vi "SRV_Motors Config GUI.vi"(11 "Motors Config File Path in":path) -> (0 "error out":errorcluster, 1 "Cancelled?":bool, 3 "Motor Config Filepath":path)   [LabVIEW 2014]
doc: "A Producer-Consumer two-loop state machine template. This template uses the LPD Command Queues to drive its execution.\n\nThere are several advantages such as:\n- convenient error state control\n- the ability to pass data between states/loops/VIs via a variant\n- command history which is extremely valuable in troubleshooting when an error occurs\n\n\nAuthor: Mike Schultz\n\nLogicPD, Inc\nwww.logicpd.com"
uses:
  SRV_Motor Control Button Config.ctl
  SRV_Motor Legos-Servo.ctl
  SRV_Motor Control Commands Cluster.ctl
  SRV_Motor Control Command Config.ctl
  SRV_Motor Control Button Icons_FALSE.ctl
  Support/SRV_Command-Data Queue Data Type.ctl
panel:
  in  "MAP":bool
  in  "Scrollbar":u32(c297)
  in  "Motor Control Config GUI":T6={"Motor Control Button Index 0"={"Button Name"="Button xx", "Button Label"="", "Motor Type"=enum."Servo", "Press Cmds"={"Motor Control Commands Array"=[]}, "Release Cmds"={"Motor Control Commands Array"=[]}, "Icon"=0}, "Motor Control Button Index 1"={"Button Name"="Button xx", "Button Label"="", "Motor Type"=enum."Servo", "Press Cmds"={"Motor Control Commands Array"=[]}, "Release Cmds"={"Motor Control Commands Array"=[]}, "Icon"=0}, "Motor Control Button Index 2"={"Button Name"="Button xx", "Button Label"="", "Motor Type"=enum."Servo", "Press Cmds"={"Motor Control Commands Array"=[]}, "Release Cmds"={"Motor Control Commands Array"=[]}, "Icon"=0}} {"Motor Control Button Index 2"."Release Cmds"."Motor Control Commands Array"."Value" format="%02x"; "Motor Control Button Index 2"."Release Cmds"."Motor Control Commands Array"."Register" format="%02x"; "Motor Control Button Index 2"."Release Cmds"."Motor Control Commands Array"."I2C Address" format="%02x"; "Motor Control Button Index 2"."Press Cmds"."Motor Control Commands Array"."Value" format="%02x"; "Motor Control Button Index 2"."Press Cmds"."Motor Control Commands Array"."Register" format="%02x"; "Motor Control Button Index 2"."Press Cmds"."Motor Control Commands Array"."I2C Address" format="%02x"; "Motor Control Button Index 1"."Release Cmds"."Motor Control Commands Array"."Value" format="%02x"; "Motor Control Button Index 1"."Release Cmds"."Motor Control Commands Array"."Register" format="%02x"; "Motor Control Button Index 1"."Release Cmds"."Motor Control Commands Array"."I2C Address" format="%02x"; "Motor Control Button Index 1"."Press Cmds"."Motor Control Commands Array"."Value" format="%02x"; "Motor Control Button Index 1"."Press Cmds"."Motor Control Commands Array"."Register" format="%02x"; "Motor Control Button Index 1"."Press Cmds"."Motor Control Commands Array"."I2C Address" format="%02x"; "Motor Control Button Index 0"."Release Cmds"."Motor Control Commands Array"."Value" format="%02x"; "Motor Control Button Index 0"."Release Cmds"."Motor Control Commands Array"."Register" format="%02x"; "Motor Control Button Index 0"."Release Cmds"."Motor Control Commands Array"."I2C Address" format="%02x"; "Motor Control Button Index 0"."Press Cmds"."Motor Control Commands Array"."Value" format="%02x"; "Motor Control Button Index 0"."Press Cmds"."Motor Control Commands Array"."Register" format="%02x"; "Motor Control Button Index 0"."Press Cmds"."Motor Control Commands Array"."I2C Address" format="%02x"}
  in  "Cancel Button":bool
  in  "OK Button":bool
  in  "About":bool
  # "I2C Address"
  # "Register"
  # "Value"
  # "Active"
  # "I2C Address"
  # "Register"
  # "Value"
  # "Active"
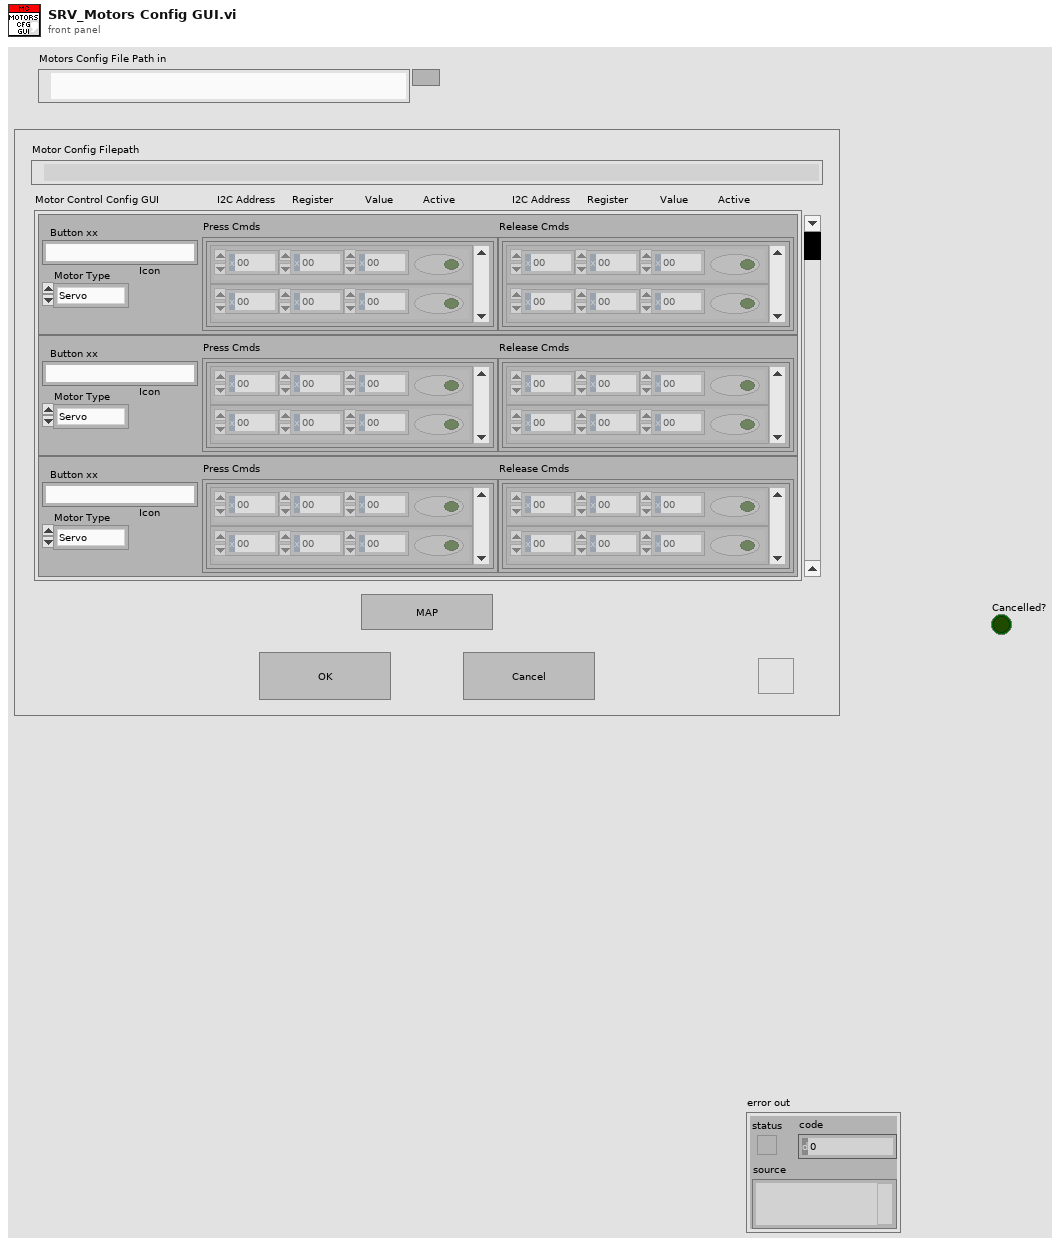
[diagram p1: front panel]
types:
  T1 = typedef "SRV_Motor Control Button Config.ctl" = cluster{"Button Name":string, "Button Label":string, "Motor Type":T2, "Press Cmds":T3, "Release Cmds":T3, "Icon":T5}
  T2 = typedef "SRV_Motor Legos-Servo.ctl" = enum16{"Servo", "Legos", "Shared Var"}
  T3 = typedef "SRV_Motor Control Commands Cluster.ctl" = cluster{"Motor Control Commands Array":T4[]}
  T4 = typedef "SRV_Motor Control Command Config.ctl" = cluster{"I2C Address":u8, "Register":u8, "Value":u8, "Active":bool}
  T5 = typedef "SRV_Motor Control Button Icons_FALSE.ctl" = u16
  T6 = cluster{"Motor Control Button Index 0":T1, "Motor Control Button Index 1":T1, "Motor Control Button Index 2":T1}
  T7 = enum8{"Enabled", "Disabled", "Disabled and Grayed Out"}
  T8 = typedef "SRV_Command-Data Queue Data Type.ctl" = cluster{"Command":string, "Data":variant}
  T9 = cluster{"user event":refnum<user-event>, "Sensor Config Filepath":path, "All Motor Control Config":T1[], "Scrollbar Value":i32, "Number Display Rows":i32, "Cancelled?":bool, "Register refs":refnum<vi>[]}
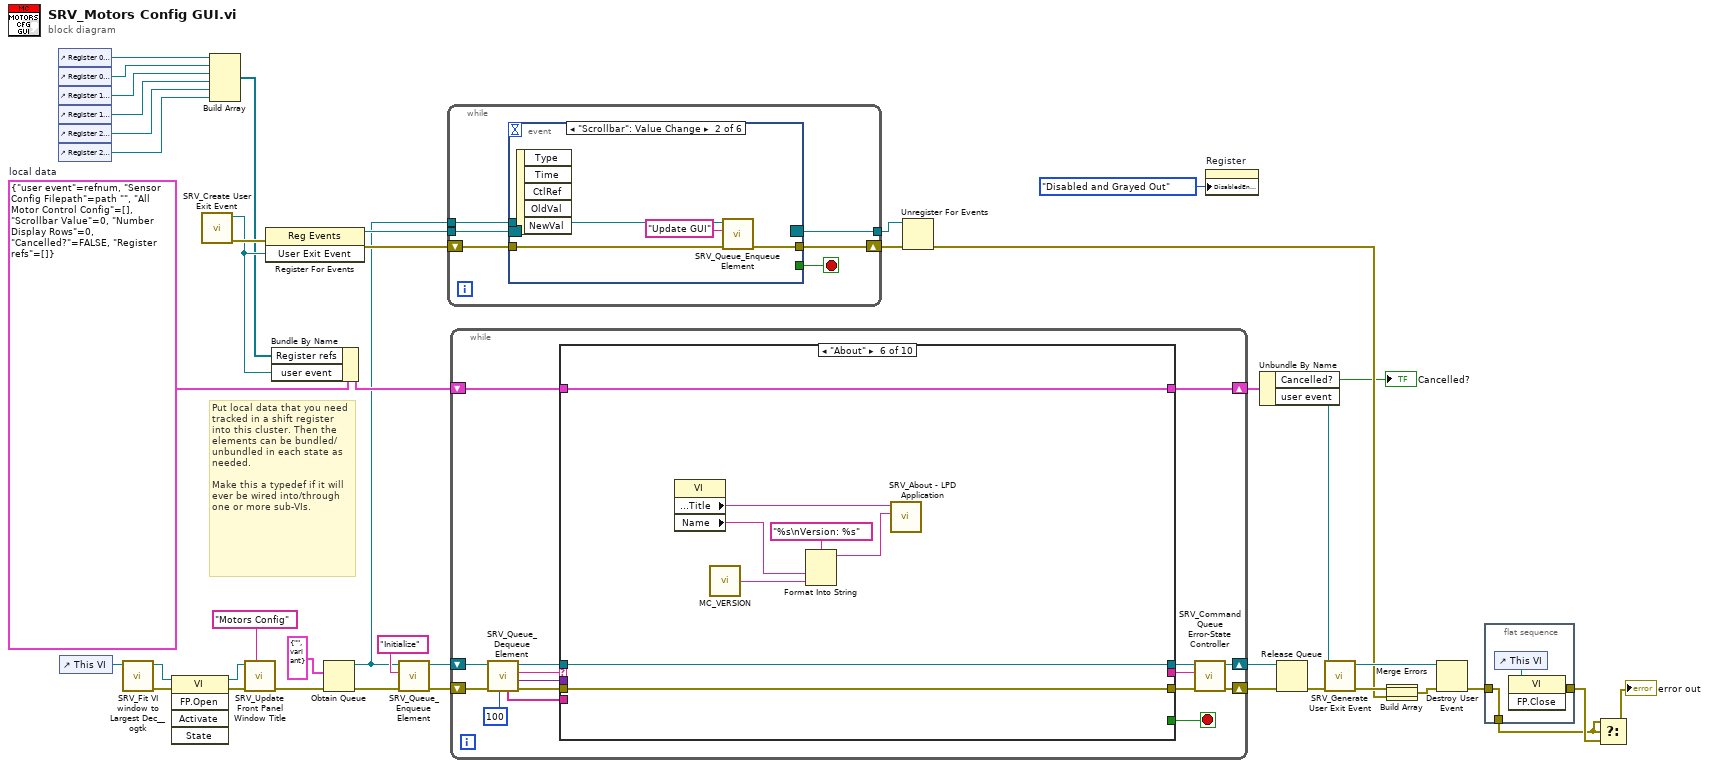
[diagram p0: block diagram]
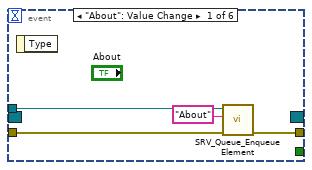
[diagram p2: hidden frame]
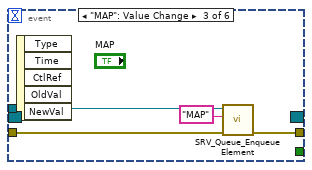
[diagram p3: hidden frame]
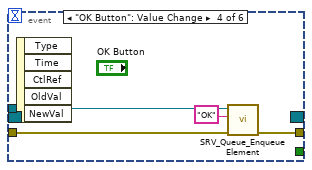
[diagram p4: hidden frame]
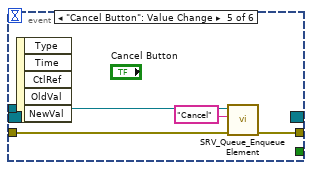
[diagram p5: hidden frame]
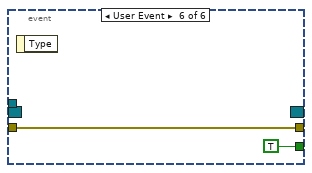
[diagram p6: hidden frame]
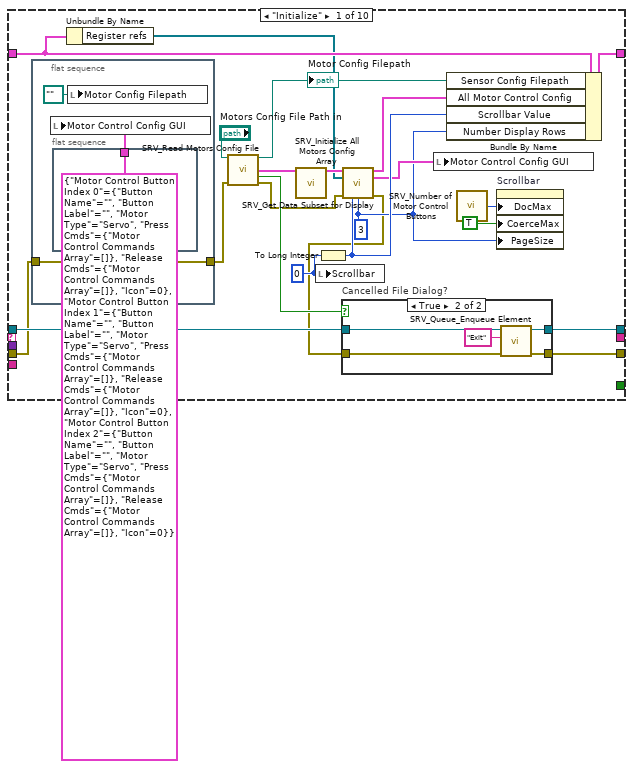
[diagram p7: hidden frame]
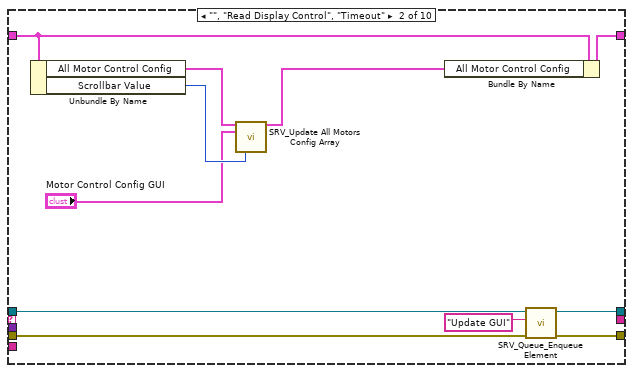
[diagram p9: hidden frame]
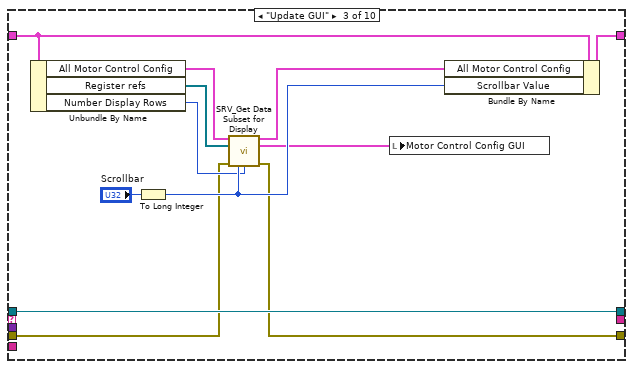
[diagram p10: hidden frame]
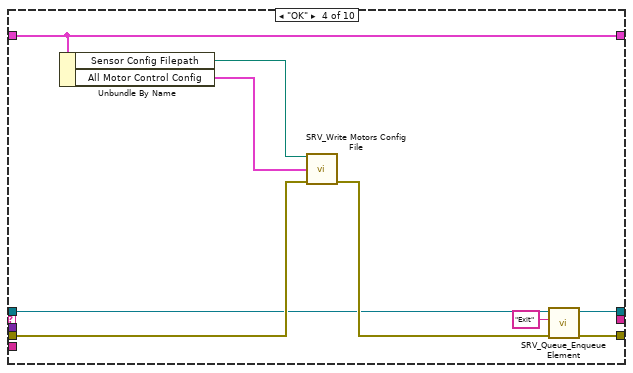
[diagram p11: hidden frame]
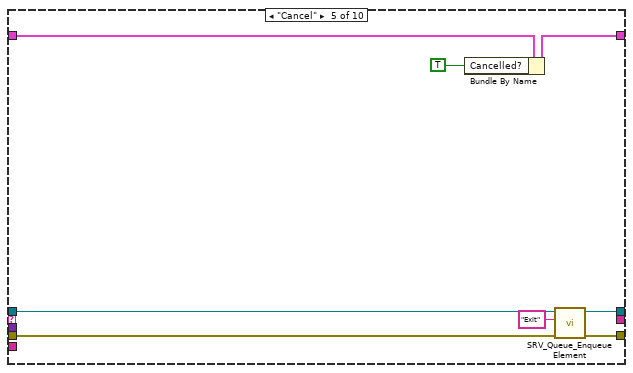
[diagram p12: hidden frame]
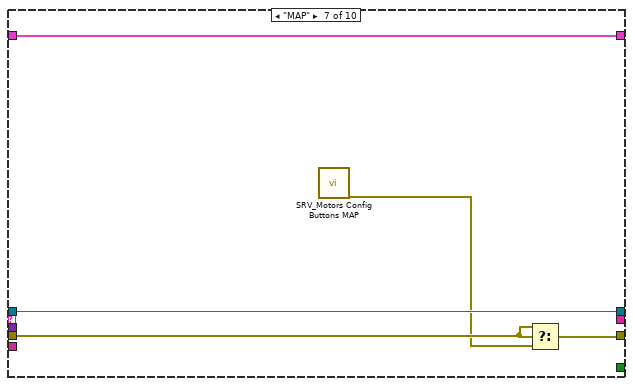
[diagram p13: hidden frame]
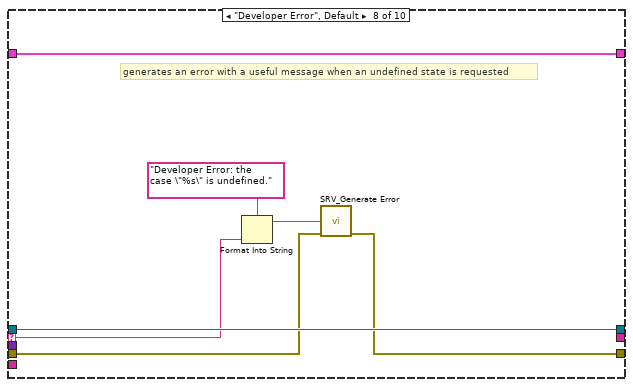
[diagram p14: hidden frame]
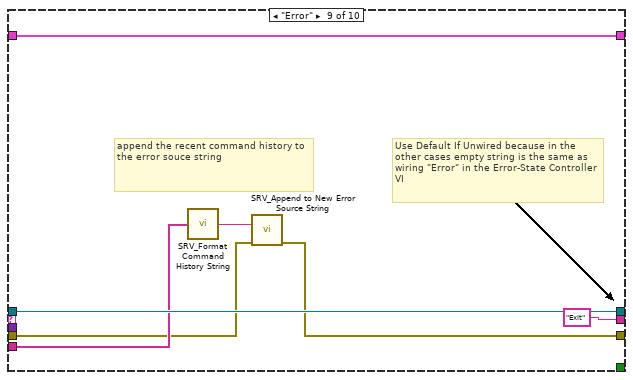
[diagram p15: hidden frame]
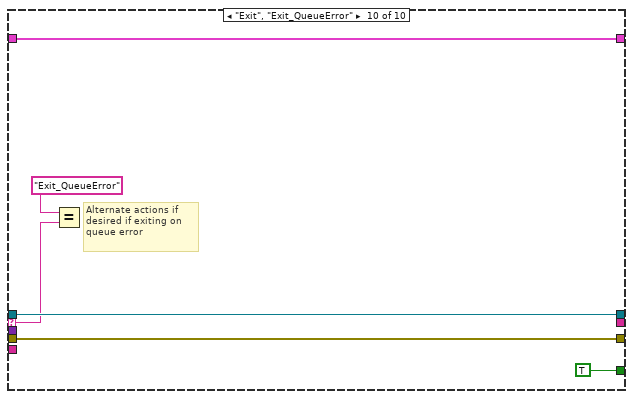
[diagram p16: hidden frame]
diagram:
  w38 = T9 {"user event"=refnum, "Sensor Config Filepath"=path "", "All Motor Control Config"=[], "Scrollbar Value"=0, "Number Display Rows"=0, "Cancelled?"=FALSE, "Register refs"=[]}  # local data
  # "Put local data that you need tracked in a shift register into this cluster. Then the elements can be bundled/unbundled in each state as needed.\n\nMake this a typedef if it will ever be wired into/through one or more sub-VIs."
  n1 = control-ref of="Register 0 Press"() -> (w7:refnum<vi>)
  n2 = control-ref of="Register 0 Release"() -> (w6:refnum<vi>)
  n3 = control-ref of="Register 1 Press"() -> (w5:refnum<vi>)
  n4 = control-ref of="Register 1 Release"() -> (w4:refnum<vi>)
  n5 = control-ref of="Register 2 Press"() -> (w3:refnum<vi>)
  n6 = control-ref of="Register 2 Release"() -> (w2:refnum<vi>)
  n7 = control-ref of="This VI"() -> (w13:refnum<vi>)
  n8 = call "SRV_Fit VI window to Largest Dec__ogtk.vi"("VI Ref (calling VI)"=w13) -> ("error out"=w16:errorcluster, "dup VI Ref"=w12:refnum<vi>)  [unwired: 5 in]
  n9 = invoke class="VI" method="FP.Open"(reference=w12, error in=w16) -> (reference out=w9:refnum<vi>, error out=w11:errorcluster)  [unwired: 3 in, 3 out]
  n10 = call "SRV_Create User Exit Event.vi"() -> ("error out"=w29:errorcluster, "User Exit Event"=w28:refnum<user-event>)  [unwired: 10 in]
  n11 = Build Array(w7, w6, w5, w4, w3, w2) -> (w1:refnum<vi>[])
  n12 = call "SRV_Update Front Panel Window Title.vi"("Window Title Override String"="Motors Config", "error in (no error)"=w11, "VI ref"=w9) -> ("error out"=w10:errorcluster)  [unwired: 7 in, 1 out]
  n13 = register-events(error in=w29, w28) -> (reference out=w44:refnum<event-registration>, error out=w43:errorcluster)  [unwired: 1 in]
  n14 = Bundle By Name(cluster=w38, "Register refs"=w1, "user event"=w28) -> (w37:T9)
  n15 = Obtain Queue(element data type=T8 {"Command"="", "Data"=variant} ("Queue Data Type"), error in (no error)=w10) -> (queue out=w24:refnum<queue>, error out=w25:errorcluster)  [unwired: 3 in, 1 out]
  n16 = call "SRV_Queue_Enqueue Element.vi"("error in (no error)"=w25, "Command"="Initialize", "Command-Data Queue"=w24) -> ("error out"=w21:errorcluster, "Command-Data Queue out"=w23:refnum<queue>)  [unwired: 6 in, 1 out]
  n17 = while {
    shift-right: [w49] -> w41
    shift-left: w43 -> [w50]
    tunnel: w24 -> [w48]
    tunnel: w44 -> [w47]
    tunnel: [w46] -> w42
    stop <- w45 stop-if-true
    n18 = event shown="[1] \"Scrollbar\": Value Change" {
      selector: w47 -> [_ _ _ _ _ _]
      dyn-events: [_ _ _ _ _ _] -> w46
      timeout: _ -> [_ _ _ _ _ _]
      tunnel: w50 -> [w54 w58 w62 w64 w68 w72]
      tunnel: [w53 w57 w61 w65 w69 w72] -> w49
      tunnel: w48 -> [w51 w55 w59 w63 w67 _]
      tunnel: [_ _ _ _ _ TRUE] -> w45
      event "About": Value Change {
        n19 = event-data() -> ()  [unwired: 1 in, 1 out]
        n20 = call "SRV_Queue_Enqueue Element.vi"("error in (no error)"=w54, "Command"="About", "Command-Data Queue"=w51) -> ("error out"=w53:errorcluster)  [unwired: 6 in, 2 out]
      }
      event "Scrollbar": Value Change {
        n21 = event-data() -> ()  [unwired: 1 in, 5 out]
        n22 = call "SRV_Queue_Enqueue Element.vi"("error in (no error)"=w58, "Command"="Update GUI", "Command-Data Queue"=w55) -> ("error out"=w57:errorcluster)  [unwired: 6 in, 2 out]
      }
      event "MAP": Value Change {
        n23 = event-data() -> ()  [unwired: 1 in, 5 out]
        n24 = call "SRV_Queue_Enqueue Element.vi"("error in (no error)"=w62, "Command"="MAP", "Command-Data Queue"=w59) -> ("error out"=w61:errorcluster)  [unwired: 6 in, 2 out]
      }
      event "OK Button": Value Change {
        n25 = event-data() -> ()  [unwired: 1 in, 5 out]
        n26 = call "SRV_Queue_Enqueue Element.vi"("error in (no error)"=w64, "Command"="OK", "Command-Data Queue"=w63) -> ("error out"=w65:errorcluster)  [unwired: 6 in, 2 out]
      }
      event "Cancel Button": Value Change {
        n27 = event-data() -> ()  [unwired: 1 in, 5 out]
        n28 = call "SRV_Queue_Enqueue Element.vi"("error in (no error)"=w68, "Command"="Cancel", "Command-Data Queue"=w67) -> ("error out"=w69:errorcluster)  [unwired: 6 in, 2 out]
      }
      event User Event {
        n29 = event-data() -> ()  [unwired: 1 in, 1 out]
      }
    }
  }
  n30 = while {
    shift-right: [w82] -> w40
    shift-left: w21 -> [w88]
    shift-right: [w80] -> w39
    shift-left: w23 -> [w86]
    shift-right: [w74] -> w36
    shift-left: w37 -> [w75]
    stop <- w76 stop-if-true
    n31 = call "SRV_Queue_Dequeue Element.vi"("timeout in ms (-1)"=100, "error in (no error)"=w88, "Command-Data Queue"=w86) -> ("error out"=w87:errorcluster, "Data"=w79:variant, "Command"=w84:string, "Command-Data Queue out"=w85:refnum<queue>, "Command History"=w78:string[])  [unwired: 3 in, 1 out]
    n32 = case shown="\"About\"" w84 {
      selector: w84 -> [_ _ _ _ _ _ _ w179 _ w191]
      tunnel: w87 -> [w103 w123 w134 w151 w160 w168 w172 w177 w183 w193]
      tunnel: [w108 w124 w133 w148 w159 w168 w171 w176 w184 w193] -> w83
      tunnel: w85 -> [w109 w126 w144 w147 w161 w169 w174 w181 w188 w194]
      tunnel: [w107 w125 w144 w146 w158 w169 w174 w181 w188 w194] -> w81
      tunnel: w79 -> [_ _ _ _ _ _ _ _ _ _]
      tunnel: w78 -> [_ _ _ _ _ _ _ _ w187 _]
      tunnel: [_ _ _ _ _ _ _ _ "Exit" ("Error Command") _] -> w77
      tunnel: [_ _ _ _ _ _ _ _ _ TRUE] -> w76
      tunnel: w75 -> [w99 w131 w142 w153 w156 w163 w173 w178 w185 w189]
      tunnel: [w106 w132 w143 w153 w155 w163 w173 w178 w185 w189] -> w74
      frame "Initialize" {
        w94 = 3 ("Number Display Rows")
        w101 = u32 0 ("Scrollbar")
        n33 = flat-sequence {
          tunnel: [w112] -> w104
          tunnel: w103 -> [w112]
          frame #0 {
            n34 = local write "Motor Control Config GUI"(w111) -> ()
            n35 = flat-sequence {
              tunnel: [T6 {"Motor Control Button Index 0"={"Button Name"="", "Button Label"="", "Motor Type"=enum."Servo", "Press Cmds"={"Motor Control Commands Array"=[]}, "Release Cmds"={"Motor Control Commands Array"=[]}, "Icon"=0}, "Motor Control Button Index 1"={"Button Name"="", "Button Label"="", "Motor Type"=enum."Servo", "Press Cmds"={"Motor Control Commands Array"=[]}, "Release Cmds"={"Motor Control Commands Array"=[]}, "Icon"=0}, "Motor Control Button Index 2"={"Button Name"="", "Button Label"="", "Motor Type"=enum."Servo", "Press Cmds"={"Motor Control Commands Array"=[]}, "Release Cmds"={"Motor Control Commands Array"=[]}, "Icon"=0}} ("Motor Control Config GUI")] -> w111
              frame #0 {
              }
            }
            n36 = local write "Motor Config Filepath"(path "" ("Sensor Config Filepath")) -> ()
          }
        }
        n37 = Unbundle By Name(w99) -> ("Register refs"=w91:refnum<vi>[])
        n38 = call "SRV_Read Motors Config File.vi"("Motors Config File Path"="Motors Config File Path in", "error in (no error)"=w104) -> ("Motors Config File Path out"=w105:path, "Motor Control Config"=w97:T1[], "Cancelled?"=w110:bool, "error out"=w90:errorcluster)  [unwired: 10 in]
        "Motor Config Filepath" <- w105
        n39 = call "SRV_Initialize All Motors Config Array.vi"("All Motor Control Config"=w97) -> ("All Motor Control Config out"=w96:T1[])  [unwired: 14 in]
        n40 = local write "Scrollbar"(w101) -> ()
        n41 = To Long Integer(number=w101) -> (32bit integer=w100:i32)
        n42 = call "SRV_Get Data Subset for Display.vi"("All Motor Control Config"=w96, "Register refs"=w91, "error in (no error)"=w90, "Row Start Index"=w100, "Number of Rows to Display (3)"=w94) -> ("All Motor Control Config dup"=w102:T1[], "Motor Control Config GUI"=w98:T6, "error out"=w89:errorcluster)  [unwired: 8 in]
        n43 = case "Cancelled File Dialog?" shown="True" w110 {
          tunnel: w89 -> [w115 w120]
          tunnel: w109 -> [w116 w121]
          tunnel: [w115 w119] -> w108
          tunnel: [w116 w118] -> w107
          frame False {
          }
          frame True {
            n44 = call "SRV_Queue_Enqueue Element.vi"("error in (no error)"=w120, "Command"="Exit", "Command-Data Queue"=w121) -> ("error out"=w119:errorcluster, "Command-Data Queue out"=w118:refnum<queue>)  [unwired: 6 in, 1 out]
          }
        }
        n45 = local write "Motor Control Config GUI"(w98) -> ()
        n46 = Bundle By Name(cluster=w99, "Sensor Config Filepath"=w105, "All Motor Control Config"=w102, "Scrollbar Value"=w100, "Number Display Rows"=w94) -> (w106:T9)
        n47 = call "SRV_Number of Motor Control Buttons.vi"() -> ("Number of Motor Control Buttons"=w92:i32)  [unwired: 14 in, 1 out]
        n48 = property on="Scrollbar" class="Scroll (strict)"("DocMax"=w92, "CoerceMax"=TRUE ("Coerce Maximum Value"), "PageSize"=w94) -> ()  [unwired: 2 in, 2 out]
      }
      frame "", "Read Display Control", "Timeout" {
        n49 = Unbundle By Name(w131) -> ("All Motor Control Config"=w128:T1[], "Scrollbar Value"=w130:i32)
        n50 = call "SRV_Update All Motors Config Array.vi"("All Motor Control Config"=w128, "Motor Control Config GUI"="Motor Control Config GUI", "Row Start Index"=w130) -> ("All Motor Control Config out"=w127:T1[])  [unwired: 12 in]
        n51 = Bundle By Name(cluster=w131, "All Motor Control Config"=w127) -> (w132:T9)
        n52 = call "SRV_Queue_Enqueue Element.vi"("error in (no error)"=w123, "Command"="Update GUI", "Command-Data Queue"=w126) -> ("error out"=w124:errorcluster, "Command-Data Queue out"=w125:refnum<queue>)  [unwired: 6 in, 1 out]
      }
      frame "Update GUI" {
        n53 = Unbundle By Name(w142) -> ("All Motor Control Config"=w139:T1[], "Register refs"=w135:refnum<vi>[], "Number Display Rows"=w136:i32)
        n54 = To Long Integer(number="Scrollbar") -> (32bit integer=w140:i32)
        n55 = call "SRV_Get Data Subset for Display.vi"("All Motor Control Config"=w139, "Register refs"=w135, "error in (no error)"=w134, "Row Start Index"=w140, "Number of Rows to Display (3)"=w136) -> ("All Motor Control Config dup"=w138:T1[], "Motor Control Config GUI"=w137:T6, "error out"=w133:errorcluster)  [unwired: 8 in]
        n56 = local write "Motor Control Config GUI"(w137) -> ()
        n57 = Bundle By Name(cluster=w142, "All Motor Control Config"=w138, "Scrollbar Value"=w140) -> (w143:T9)
      }
      frame "OK" {
        n58 = Unbundle By Name(w153) -> ("Sensor Config Filepath"=w152:path, "All Motor Control Config"=w145:T1[])
        n59 = call "SRV_Write Motors Config File.vi"("Motors Config File Path"=w152, "Motor Control Config"=w145, "error in (no error)"=w151) -> ("error out"=w149:errorcluster)  [unwired: 12 in]
        n60 = call "SRV_Queue_Enqueue Element.vi"("error in (no error)"=w149, "Command"="Exit", "Command-Data Queue"=w147) -> ("error out"=w148:errorcluster, "Command-Data Queue out"=w146:refnum<queue>)  [unwired: 6 in, 1 out]
      }
      frame "Cancel" {
        n61 = Bundle By Name(cluster=w156, "Cancelled?"=TRUE) -> (w155:T9)
        n62 = call "SRV_Queue_Enqueue Element.vi"("error in (no error)"=w160, "Command"="Exit", "Command-Data Queue"=w161) -> ("error out"=w159:errorcluster, "Command-Data Queue out"=w158:refnum<queue>)  [unwired: 6 in, 1 out]
      }
      frame "About" {
        n63 = property class="VI"() -> ("Front Panel.Title"=w167:string, "Name"=w164:string)  [unwired: 2 in, 2 out]
        n64 = call "MC_VERSION.vi"() -> ("MC Version"=w162:string)
        n65 = Format Into String(format string="%s\nVersion: %s", w164, w162) -> (resulting string=w165:string)  [unwired: 2 in, 1 out]
        n66 = call "SRV_About - LPD Application.vi"("Version Info"=w165, "Application Name"=w167) -> ()  [unwired: 10 in]
      }
      frame "MAP" {
        n67 = call "SRV_Motors Config Buttons MAP.vi"() -> ("error out"=w170:errorcluster)  [unwired: 11 in]
        n68 = Select(t=w172, s=w172, f=w170) -> (s? t:f=w171:errorcluster)
      }
      frame "Developer Error", Default {
        # "generates an error with a useful message when an undefined state is requested"
        n69 = Format Into String(format string="Developer Error: the case \"%s\" is undefined.", w179) -> (resulting string=w175:string)  [unwired: 2 in, 1 out]
        n70 = call "SRV_Generate Error.vi"("Message"=w175, "error in (no error)"=w177) -> ("error out"=w176:errorcluster)  [unwired: 13 in]
      }
      frame "Error" {
        # "Use Default If Unwired because in the other cases empty string is the same as wiring \"Error\" in the Error-State Controller VI"
        # "append the recent command history to the error souce string"
        n71 = call "SRV_Format Command History String.vi"("Command History"=w187) -> ("Command History String"=w182:string)  [unwired: 14 in]
        n72 = call "SRV_Append to New Error Source String.vi"("Message String to append"=w182, "Error In (no error)"=w183) -> ("error out"=w184:errorcluster)  [unwired: 13 in]
      }
      frame "Exit", "Exit_QueueError" {
        # "Alternate actions if desired if exiting on queue error"
        n73 = Equal?(x="Exit_QueueError", y=w191) -> ()  [unwired: 1 out]
      }
    }
    n74 = call "SRV_Command Queue Error-State Controller.vi"("error in (no error)"=w83, "Error Command"=w77, "Command-Data Queue"=w81) -> ("error out"=w82:errorcluster, "Command-Data Queue out"=w80:refnum<queue>)  [unwired: 7 in]
  }
  n75 = Unregister For Events(event registration refnum=w42, error in=w41) -> (error out=w31:errorcluster)
  n76 = property on="Register" class="DigNum (strict)"("DisabledEnum"=T7."Disabled and Grayed Out" ("Disabled")) -> ()  [unwired: 2 in, 2 out]
  n77 = Unbundle By Name(w36) -> ("Cancelled?"=→"Cancelled?":bool, "user event"=w35:refnum<user-event>)
  n78 = Release Queue(queue=w39, error in (no error)=w40) -> (error out=w34:errorcluster)  [unwired: 1 in, 2 out]
  n79 = call "SRV_Generate User Exit Event.vi"("error in (no error)"=w34, "User Exit Event"=w35) -> ("error out"=w32:errorcluster, "User Exit Event out"=w33:refnum<user-event>)  [unwired: 8 in]
  n80 = Build Array(w32, w31) -> (w27:errorcluster[])
  n81 = Merge Errors(w27) -> (w30:errorcluster)
  n82 = Destroy User Event(user event=w33, error in=w30) -> (error out=w18:errorcluster)
  n83 = flat-sequence {
    tunnel: [w196] -> w20
    tunnel: w18 -> [w195]
    tunnel: [w195] -> w17
    frame #0 {
      n84 = control-ref of="This VI"() -> (w197:refnum<vi>)
      n85 = invoke class="VI" method="FP.Close"(reference=w197) -> (error out=w196:errorcluster)  [unwired: 2 in, 2 out]
    }
  }
  n86 = Select(t=w17, s=w17, f=w20) -> (s? t:f=→"error out":errorcluster)
